vi "MongoDB.EnsureIndex.vi"(8 "error in (no error)":errorcluster, 11 "MongoDB.Collection in":refnum<class "MongoDB.Collection.lvclass">) -> (0 "error out":errorcluster, 3 "MongoDB.Collection out":refnum<class "MongoDB.Collection.lvclass">)   [LabVIEW 2014, in "MongoDB.Collection.lvclass"]
uses:
  MongoDB.Collection.lvclass
  MongoDB.Collection.lvclass/MongoDB.Collection.ctl
  C:/Users/Richard/Documents/GitHub/mongo-labview-driver/CSharp/bin/MongoDB.Driver.Legacy.dll
  CSharp/bin/MongoDB.Driver.Legacy.dll
panel:
  out "keyNames out":string[](array[string])
  in  "keyNames":string[](array[string])
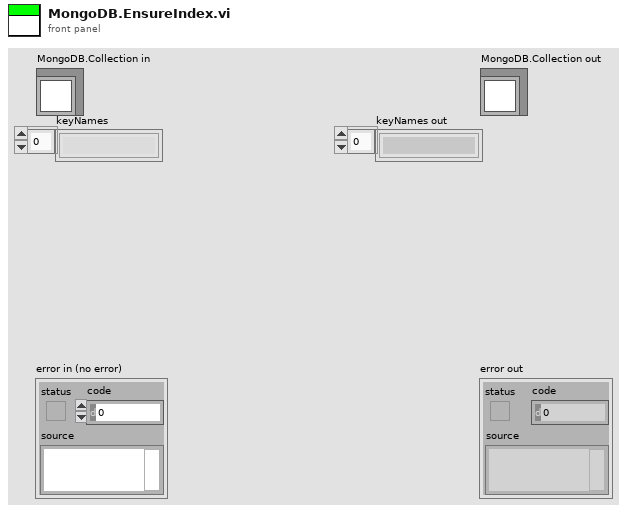
[diagram p1: front panel]
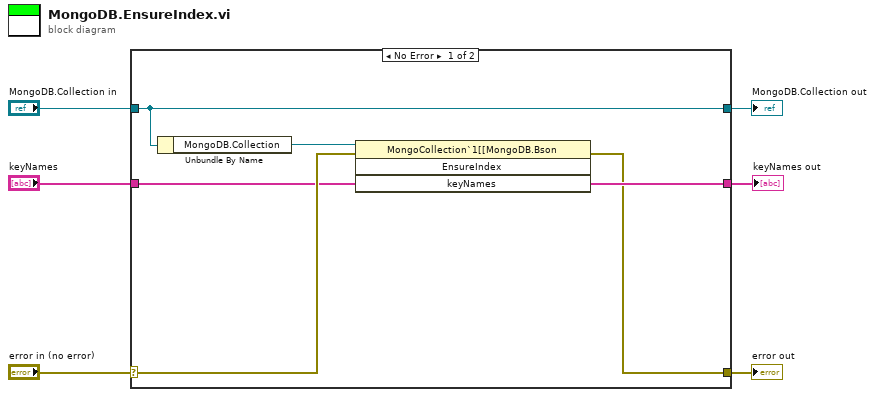
[diagram p0: block diagram]
diagram:
  n1 = case shown="No Error" "error in (no error)" {
    selector: "error in (no error)" -> [w10 w15]
    tunnel: [w7 w15] -> w5
    tunnel: [w12 w14] -> w3
    tunnel: "MongoDB.Collection in" -> [w12 w14]
    tunnel: "keyNames" -> [w9 w13]
    tunnel: [w8 w13] -> w1
    frame No Error {
      n2 = Unbundle By Name(w12) -> ("MongoDB.Collection"=w11:refnum<k24>)
      n3 = invoke class="MongoCollection`1[[MongoDB.Bson" method="EnsureIndex"(reference=w11, error in=w10, "keyNames"=w9) -> (error out=w7:errorcluster, "keyNames"=w8:string[])  [unwired: 1 in, 2 out]
    }
    frame Error {
    }
  }
  "error out" <- w5
  "MongoDB.Collection out" <- w3
  "keyNames out" <- w1
